vi "Select DMM voltage range.vi"(8 "error in (no error)":errorcluster, 11 "Max":dbl) -> (0 "error out":errorcluster, 3 "DDM voltage Range":dbl)   [LabVIEW 2018, in "Application.lvlib"]
uses:
  Application.lvlib
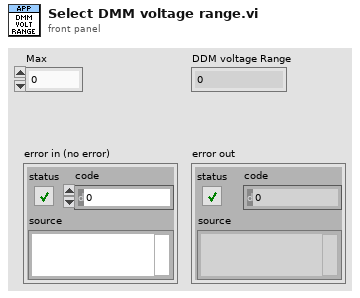
[diagram p1: front panel]
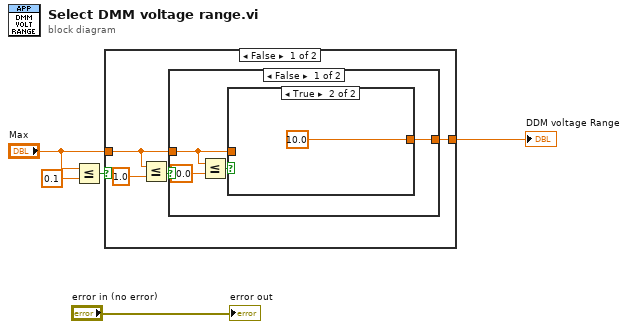
[diagram p0: block diagram]
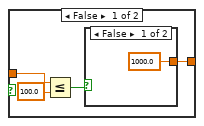
[diagram p2: hidden frame]
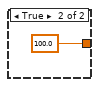
[diagram p3: hidden frame]
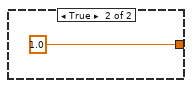
[diagram p4: hidden frame]
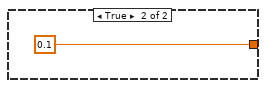
[diagram p5: hidden frame]
diagram:
  n1 = Less Or Equal?(x="Max", y=0.1) -> (x <= y?=w3:bool)
  n2 = case shown="False" w3 {
    tunnel: [w7 0.1] -> w2
    tunnel: "Max" -> [w6 _]
    frame False {
      n3 = Less Or Equal?(x=w6, y=1.0) -> (x <= y?=w8:bool)
      n4 = case shown="False" w8 {
        tunnel: [w11 1.0 ("y")] -> w7
        tunnel: w6 -> [w10 _]
        frame False {
          n5 = Less Or Equal?(x=w10, y=10.0) -> (x <= y?=w12:bool)
          n6 = case shown="True" w12 {
            tunnel: [w14 10.0] -> w11
            tunnel: w10 -> [w17 _]
            frame False {
              n7 = Less Or Equal?(x=w17, y=100.0) -> (x <= y?=w15:bool)
              n8 = case shown="False" w15 {
                tunnel: [1000.0 100.0] -> w14
                frame False {
                }
                frame True {
                }
              }
            }
            frame True {
            }
          }
        }
        frame True {
        }
      }
    }
    frame True {
    }
  }
  "DDM voltage Range" <- w2
  "error out" <- "error in (no error)"
